vi "PF fenli.vi"(10 "连板数":i32=4, 11 "PF":string[][](array[string])) -> (2 "board PF":bool[](array[boolean]))   [LabVIEW 2018]
panel:
  in  "TEST":i32(listbox)
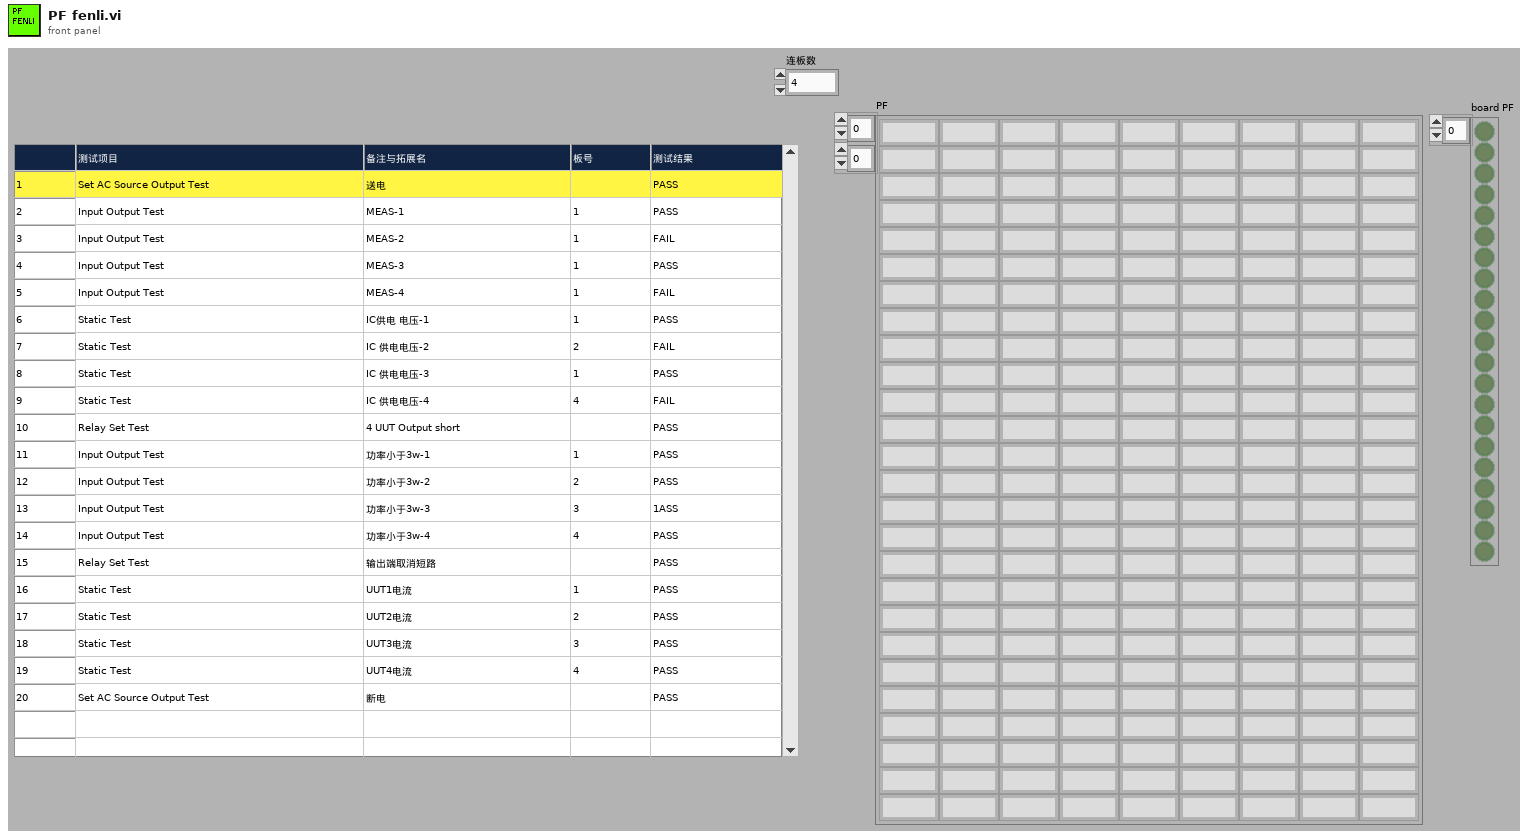
[diagram p1: front panel]
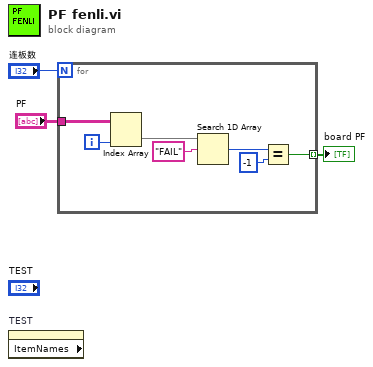
[diagram p0: block diagram]
diagram:
  n1 = property on="TEST" class="MCListbox (严格)" props=["ItemNames"]() -> ()  [unwired: 2 in, 3 out]
  n2 = for {
    N: "连板数" -> [_]
    tunnel: "PF" -> [w8]
    tunnel: [w7] -> w2 mode=indexing
    i -> [w10]
    n3 = Index Array(array=w8, index (col)=w10) -> (element=w9:string[])  [unwired: 1 in]
    n4 = Search 1D Array(1D array=w9, element="FAIL" ("元素")) -> (index of element=w5:i32)  [unwired: 1 in]
    n5 = Equal?(x=w5, y=-1) -> (x = y?=w7:bool)
  }
  "board PF" <- w2
